vi "Method String Input.vi"(8 "error in (no error)":errorcluster, 10 "String Input":string, 11 "Test Interface Mock In":refnum<class "Test Interface Mock.lvclass">) -> (0 "error out":errorcluster, 3 "Test Interface Mock Out":refnum<class "Test Interface Mock.lvclass">)   [LabVIEW 2020, in "Test Interface Mock.lvclass"]
uses:
  Test Interface Mock.lvclass
  Test Interface Mock.lvclass/Test Interface Mock.ctl
  source/Framework/Mock/Mock.lvclass
  C:/git/astemes-lmock/source/Framework/Mock/Mock.lvclass
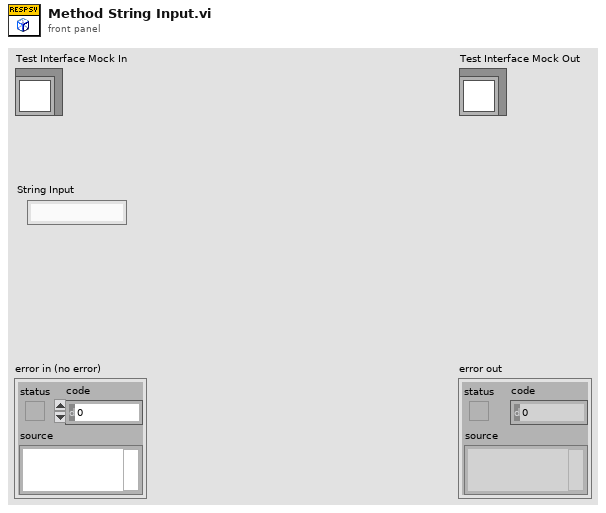
[diagram p1: front panel]
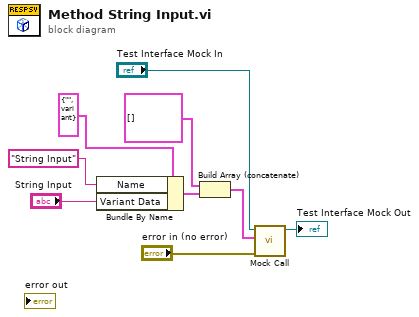
[diagram p0: block diagram]
diagram:
  n1 = Bundle By Name(cluster=cluster{"Name":string, "Variant Data":variant} {"Name"="", "Variant Data"=variant} ("element"), "Name"="String Input", "Variant Data"="String Input") -> (w1:cluster{"Name":string, "Variant Data":variant})
  n2 = Build Array (concatenate)(cluster{"Name":string, "Variant Data":variant}[] [] ("Control Values"), w1) -> (w5:cluster{"Name":string, "Variant Data":variant}[])
  n3 = call "Mock Call.vi"("error in (no error)"="error in (no error)", "Control Values"=w5, "Mock In"="Test Interface Mock In") -> ("Mock Out"=→"Test Interface Mock Out":refnum<class "Test Interface Mock.lvclass">)  [unwired: 7 in, 1 out]
